vi "Format.vi"(6 "Statement":T1={"timestamp"=timestamp(0 s since 1904-01-01), "level"=enum."INFO", "sourceTag"="", "originVI"="", "message"=""}, 8 "error in (no error)":errorcluster, 11 "TextLayout in":refnum<class "TextLayout.lvclass">) -> (0 "error out":errorcluster, 3 "TextLayout out":refnum<class "TextLayout.lvclass">, 4 "FormattedLine":string)   [LabVIEW 2026, in "Lumberjack.lvlib" / "TextLayout.lvclass"]
doc: "Override of Layout:Format. Compose a readable line from the Statement (e.g. \"timestamp level [sourceTag] message\"); no strict quoting.\n\nTip: Emit a readable single line from a Statement."
uses:
  TextLayout.lvclass
  TypeDefs/Statement.ctl
  TypeDefs/Severity.ctl
  TextLayout.lvclass/TextLayout.ctl
  Layout.lvclass/Layout.lvclass
  Lumberjack.lvlib
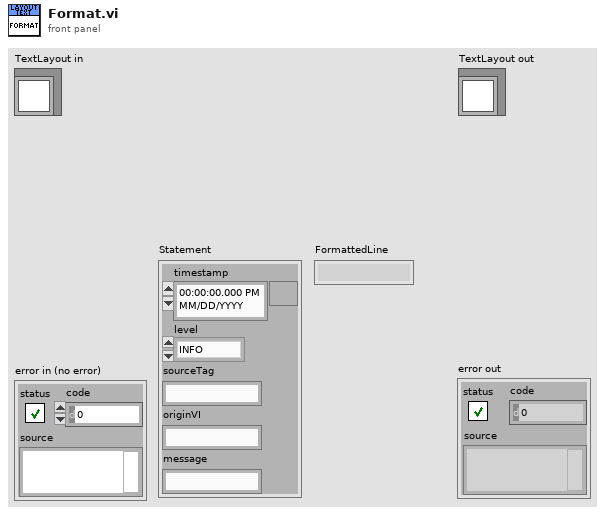
[diagram p1: front panel]
types:
  T1 = typedef "Lumberjack.lvlib/Statement.ctl" = cluster{"timestamp":timestamp, "level":T2, "sourceTag":string, "originVI":string, "message":string}
  T2 = typedef "Lumberjack.lvlib/Severity.ctl" = enum16{"OFF", "FATAL", "ERROR", "WARN", "INFO", "DEBUG", "TRACE", "ALL"}
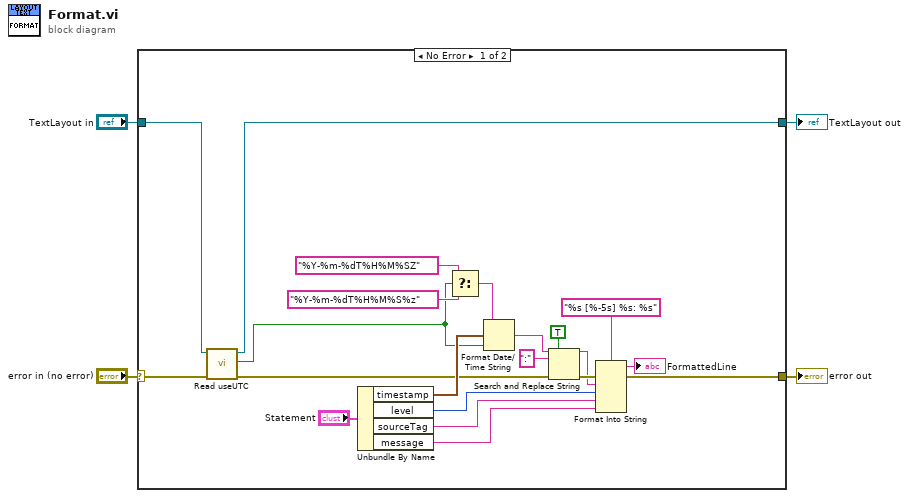
[diagram p0: block diagram]
diagram:
  n1 = case shown="No Error" "error in (no error)" {
    selector: "error in (no error)" -> [w16 w26]
    tunnel: [w11 w26] -> w4
    tunnel: [w15 w27] -> w3
    tunnel: "TextLayout in" -> [w17 w27]
    frame No Error {
      n2 = call "Read useUTC.vi"("error in (no error)"=w16, "Layout in"=w17) -> ("error out"=w5:errorcluster, "useUTC"=w14:bool, "Layout out"=w15:refnum<class "TextLayout.lvclass">)  [unwired: 7 in]
      n3 = Unbundle By Name("Statement") -> ("timestamp"=w18:timestamp, "level"=w6:T2, "sourceTag"=w9:string, "message"=w8:string)
      n4 = Select(t="%Y-%m-%dT%H%M%SZ" ("time format string (%c)"), s=w14, f="%Y-%m-%dT%H%M%S%z" ("time format string (%c)")) -> (s? t:f=w23:string)
      n5 = Format Date/Time String(time format string (%c)=w23, seconds (now)=w18, UTC format=w14) -> (date/time string=w21:string)
      n6 = Search and Replace String(replace all?=TRUE ("replace all? (F)"), input string=w21, search string=":", error in=w5) -> (result string=w10:string, error out=w12:errorcluster)  [unwired: 4 in, 2 out]
      n7 = Format Into String(format string="%s [%-5s] %s: %s", error in=w12, w10, w6, w9, w8) -> (resulting string=→"FormattedLine":string, error out=w11:errorcluster)  [unwired: 1 in]
    }
    frame Error {
    }
  }
  "error out" <- w4
  "TextLayout out" <- w3
